vi "Write Device Configurations.vi"(8 "error in (no error)":errorcluster, 10 "Device Configurations":T1={"Trace Config"={"Trace Selection"=enum."Trace A", "Roll Avg"=2.0}, "Measurement Config"={"Wavelength"={"Center Wavelength (nm)"=1550.0, "Span (nm)"=10.0}, "Sampling"={"Mode"=enum."Auto", "No. Samples"=5501}, "Sens-Resolution"={"Resolution (nm)"=0.0}, "Main Scale"={"Reference Level (dBm)"=0.0, "Log Scale (dB/Div)"=0.0}}}, 11 "Optical Spectrum Analyzer in":refnum<class "Optical Spectrum Analyzer.lvclass">) -> (0 "error out":errorcluster, 3 "Optical Spectrum Analyzer out":refnum<class "Optical Spectrum Analyzer.lvclass">)   [LabVIEW 2018, in "Optical Spectrum Analyzer.lvlib" / "Optical Spectrum Analyzer.lvclass"]
uses:
  Optical Spectrum Analyzer.lvclass
  Custom Controls/cls_Device Configurations.ctl
  Custom Controls/enm_Trace Selection.ctl
  Optical Spectrum Analyzer.lvclass/Optical Spectrum Analyzer.ctl
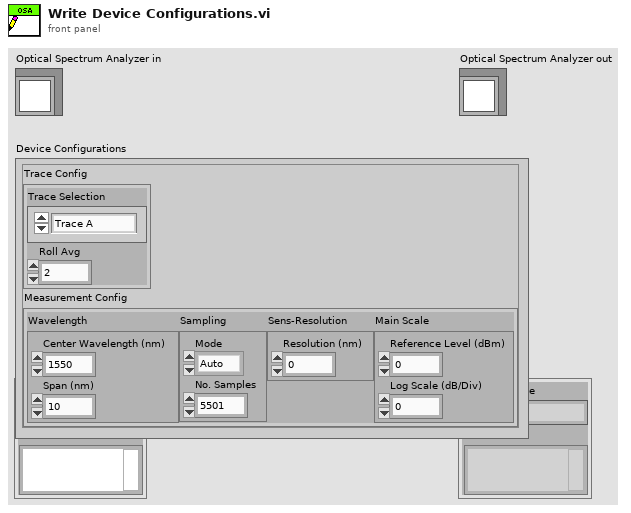
[diagram p1: front panel]
types:
  T1 = typedef "Optical Spectrum Analyzer.lvlib/Optical Spectrum Analyzer.lvclass/cls_Device Configurations.ctl" = cluster{"Trace Config":cluster{"Trace Selection":T2, "Roll Avg":dbl}, "Measurement Config":cluster{"Wavelength":cluster{"Center Wavelength (nm)":dbl, "Span (nm)":dbl}, "Sampling":cluster{"Mode":enum16{"Auto", "Manual"}, "No. Samples":u32}, "Sens-Resolution":cluster{"Resolution (nm)":dbl}, "Main Scale":cluster{"Reference Level (dBm)":dbl, "Log Scale (dB/Div)":dbl}}}
  T2 = typedef "Optical Spectrum Analyzer.lvlib/Optical Spectrum Analyzer.lvclass/enm_Trace Selection.ctl" = enum16{"Trace A", "Trace B", "Trace C", "Trace D", "Trace E", "Trace F", "Trace G"}
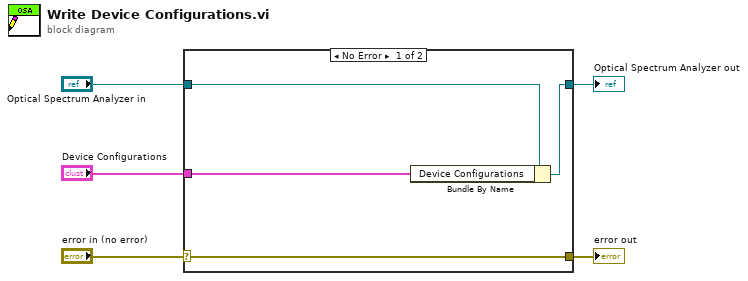
[diagram p0: block diagram]
diagram:
  n1 = case shown="No Error" "error in (no error)" {
    selector: "error in (no error)" -> [w9 w10]
    tunnel: [w9 w10] -> w4
    tunnel: [w7 w11] -> w2
    tunnel: "Optical Spectrum Analyzer in" -> [w8 w11]
    tunnel: "Device Configurations" -> [w6 _]
    frame No Error {
      n2 = Bundle By Name(cluster=w8, "Device Configurations"=w6) -> (w7:refnum<class "Optical Spectrum Analyzer.lvclass">)
    }
    frame Error {
    }
  }
  "error out" <- w4
  "Optical Spectrum Analyzer out" <- w2
